vi "Update Current Tool.vi"(8 "error in (no error)":errorcluster, 10 "Tool Buttons":T1, 11 "Map Model in":refnum<class "Map Model.lvclass">) -> (0 "error out":errorcluster, 3 "Map Model out":refnum<class "Map Model.lvclass">)   [LabVIEW 2020, in "Map Model.lvlib" / "Map Model.lvclass"]
uses:
  Map Model.lvclass
  Type Definitions/Tool Buttons.ctl
  Map Model.lvclass/Map Model.ctl
panel:
  # "NOTICE -- YOU MUST LEAVE THIS NOTICE IN PLACE.\n\nCopyright (c) 2017, LIANG LIU Shawn.Liu.cn@gmail.com\nAll rights reserved.\n\nRedistribution and use in source and binary forms, with or without modification, are permitted provided that the following conditions are met:\n-Redistributions of source code must retain the above copyright notice, this list of conditions and the following disclaimer.\n-Redistributions in binary form must reproduce the above copyright notice, this list of conditions and the following disclaimer in the documentation and/or other materials provided with the distribution.\n-Neither the name of the eLp nor the names of its contributors may be used to endorse or promote products derived from this software without specific prior written permission.\n\nTHIS SOFTWARE IS PROVIDED BY THE COPYRIGHT HOLDERS AND CONTRIBUTORS \"AS IS\" AND ANY EXPRESS OR IMPLIED WARRANTIES, INCLUDING, BUT NOT LIMITED TO, THE IMPLIED WARRANTIES OF MERCHANTABILITY AND FITNESS FOR A PARTICULAR PURPOSE ARE DISCLAIMED. IN NO EVENT SHALL THE COPYRIGHT HOLDER OR CONTRIBUTORS BE LIABLE FOR ANY DIRECT, INDIRECT, INCIDENTAL, SPECIAL, EXEMPLARY, OR CONSEQUENTIAL DAMAGES (INCLUDING, BUT NOT LIMITED TO, PROCUREMENT OF SUBSTITUTE GOODS OR SERVICES; LOSS OF USE, DATA, OR PROFITS; OR BUSINESS INTERRUPTION) HOWEVER CAUSED AND ON ANY THEORY OF LIABILITY, WHETHER IN CONTRACT, STRICT LIABILITY, OR TORT (INCLUDING NEGLIGENCE OR OTHERWISE) ARISING IN ANY WAY OUT OF THE USE OF THIS SOFTWARE, EVEN IF ADVISED OF THE POSSIBILITY OF SUCH DAMAGE."
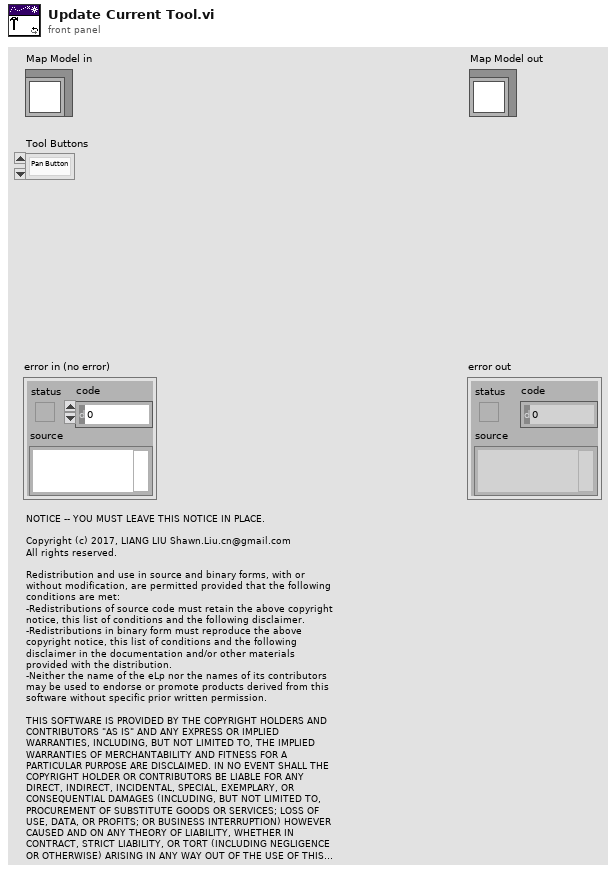
[diagram p1: front panel]
types:
  T1 = typedef "Tool Buttons.ctl" = enum32{"Pan Button", "Pencil Button", "Line Button", "Eraser Button", "Rectangle Select Button", "Deselect Button", "Crop Button", "Rotate Button", "Set Origin Button", "Zoom In Button", "Zoom Out Button"}
  T2 = enum8{"Enabled", "Disabled", "Disabled and Grayed Out"}
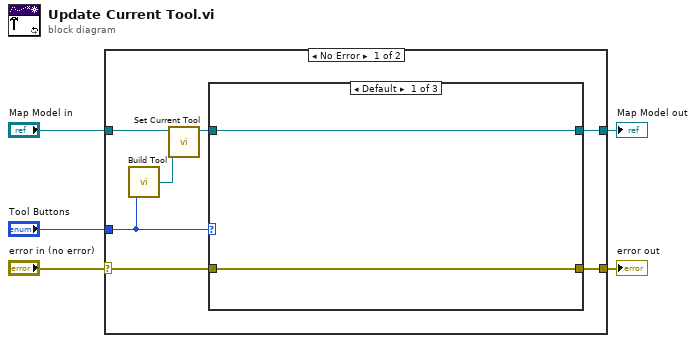
[diagram p0: block diagram]
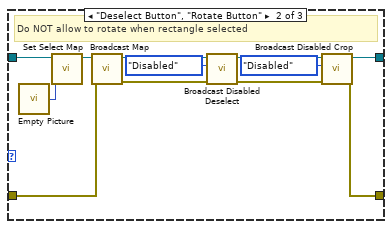
[diagram p2: hidden frame]
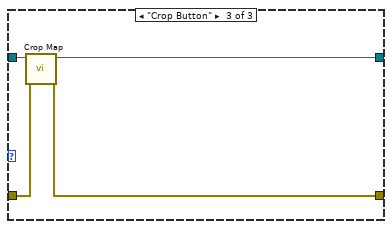
[diagram p3: hidden frame]
diagram:
  n1 = case shown="No Error" "error in (no error)" {
    selector: "error in (no error)" -> [w7 w32]
    tunnel: "Map Model in" -> [w12 w31]
    tunnel: "Tool Buttons" -> [w9 _]
    tunnel: [w8 w31] -> w3
    tunnel: [w6 w32] -> w1
    frame No Error {
      n2 = call "Build Tool.vi"("Tool Buttons"=w9) -> ("Tool"=w11:refnum<class "Tool.lvclass">)
      n3 = call "Set Current Tool.vi"("Current Tool"=w11, "Map Model in"=w12) -> ("Map Model out"=w10:refnum<class "Map Model.lvclass">)  [unwired: 9 in]
      n4 = case shown="Default" w9 {
        tunnel: w10 -> [w14 w26 w30]
        tunnel: [w14 w20 w29] -> w8
        tunnel: w7 -> [w13 w22 w28]
        tunnel: [w13 w15 w27] -> w6
        frame Default {
        }
        frame "Deselect Button", "Rotate Button" {
          # "Do NOT allow to rotate when rectangle selected"
          n5 = call "Empty Picture"() -> ("empty picture"=w24:picture)
          n6 = call "Set Select Map.vi"("Select Map"=w24, "Map Model in"=w26) -> ("Map Model out"=w25:refnum<class "Map Model.lvclass">)  [unwired: 9 in]
          n7 = call "Broadcast Map.vi"("error in (no error)"=w22, "Map Model in"=w25) -> ("error out"=w17:errorcluster, "Map Model out"=w23:refnum<class "Map Model.lvclass">)  [unwired: 8 in]
          n8 = call "Broadcast Disabled Deselect.vi"("error in (no error)"=w17, "Disabled Deselect"=T2."Disabled", "Map Model in"=w23) -> ("error out"=w16:errorcluster, "Map Model out"=w21:refnum<class "Map Model.lvclass">)  [unwired: 7 in]
          n9 = call "Broadcast Disabled Crop.vi"("error in (no error)"=w16, "Disabled Crop"=T2."Disabled", "Map Model in"=w21) -> ("error out"=w15:errorcluster, "Map Model out"=w20:refnum<class "Map Model.lvclass">)  [unwired: 7 in]
        }
        frame "Crop Button" {
          n10 = call "Crop Map.vi"("error in (no error)"=w28, "Map Model in"=w30) -> ("error out"=w27:errorcluster, "Map Model out"=w29:refnum<class "Map Model.lvclass">)  [unwired: 8 in]
        }
      }
    }
    frame Error {
    }
  }
  "error out" <- w1
  "Map Model out" <- w3
